vi "SCMP - rot180 array.vi"(7 "pic op (noop)":enum16{"noop", "Rot180", "Flip180"}(ring), 11 "A in":u32[][](array[numeric])) -> (3 "A out":u32[][](array[numeric]))   [LabVIEW 2014]
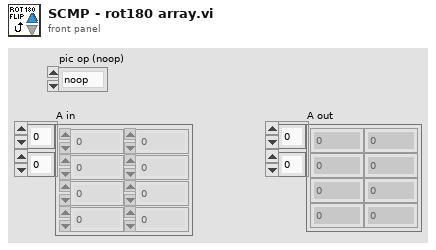
[diagram p1: front panel]
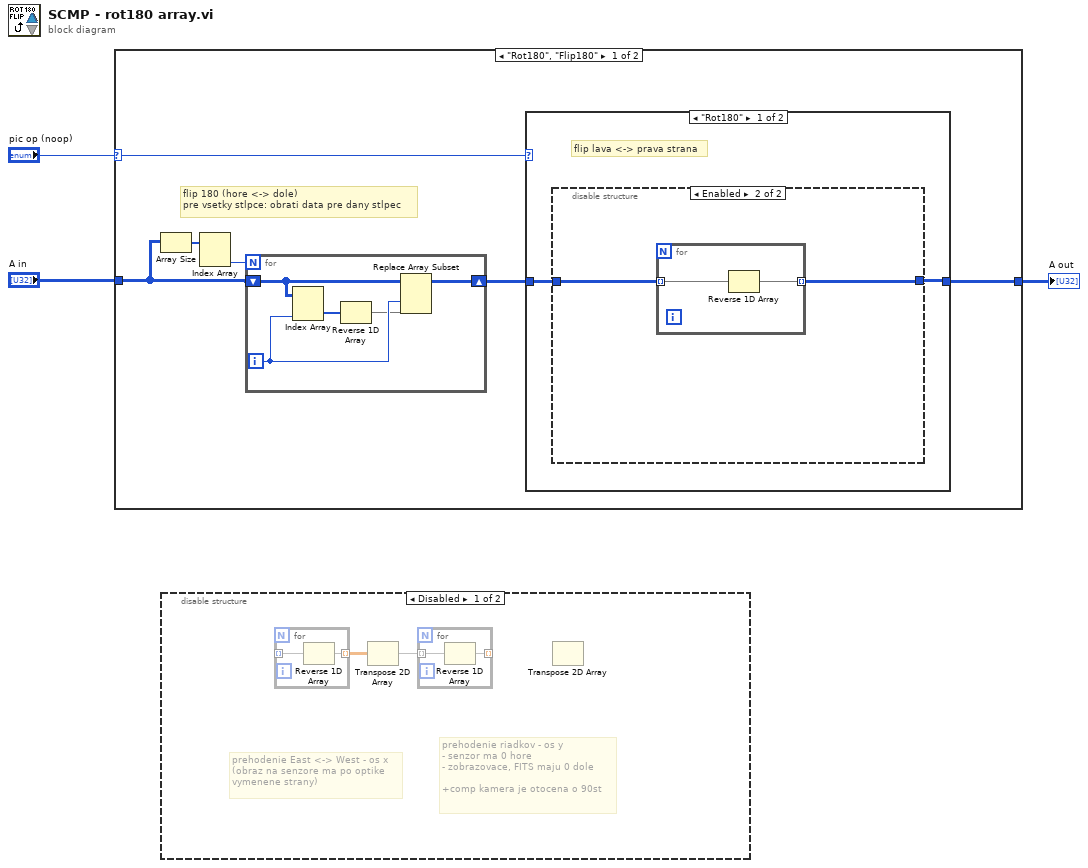
[diagram p0: block diagram]
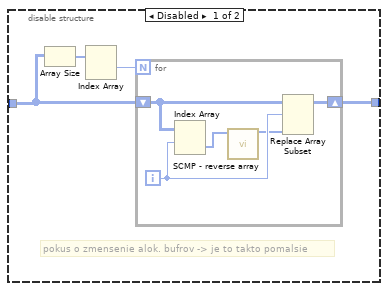
[diagram p3: hidden frame]
diagram:
  n1 = case shown="\"Rot180\", \"Flip180\"" "pic op (noop)" {
    selector: "pic op (noop)" -> [w5 _]
    tunnel: "A in" -> [w9 w31]
    tunnel: [w4 w31] -> w2
    frame "Rot180", "Flip180" {
      # "flip 180 (hore <-> dole)\npre vsetky stlpce: obrati data pre dany stlpec"
      n2 = Array Size(array=w9) -> (size(s)=w7:i32[])
      n3 = Index Array(array=w7) -> (element #2=w8:i32)  [unwired: 2 in, 1 out]
      n4 = for {
        N: w8 -> [_]
        shift-right: [w29] -> w6
        shift-left: w9 -> [w28]
        i -> [w30]
        n5 = Index Array(array=w28, index (col)=w30) -> (element=w27:u32[])  [unwired: 1 in]
        n6 = Reverse 1D Array(array=w27) -> (reversed array=w26:u32[])
        n7 = Replace Array Subset(array=w28, new element=w26, index (col)=w30) -> (w29:u32[][])  [unwired: 1 in]
      }
      n8 = case shown="\"Rot180\"" w5 {
        tunnel: w6 -> [w10 w25]
        tunnel: [w11 w25] -> w4
        frame "Rot180" {
          # "flip lava <-> prava strana"
          n9 = disable-structure shown="Enabled" {
            disable-tunnel: [w13 w21] -> w11
            disable-tunnel: w10 -> [w12 w22]
            frame Disabled {
              # "pokus o zmensenie alok. bufrov -> je to takto pomalsie"
              n10 = Array Size(array=w12) -> (size(s)=w15:i32[])
              n11 = Index Array(array=w15) -> (element #1=w14:i32)  [unwired: 2 in, 1 out]
              n12 = for {
                N: w14 -> [_]
                shift-right: [w19] -> w13
                shift-left: w12 -> [w18]
                i -> [w17]
                n13 = Index Array(array=w18, index (row)=w17) -> (element=w20:u32[])  [unwired: 1 in]
                n14 = call "SCMP - reverse array.vi"("A in"=w20) -> ("Array"=w16:u16[])  [unwired: 10 in]
                n15 = Replace Array Subset(array=w18, new element=w16, index (row)=w17) -> (w19:u32[][])  [unwired: 1 in]
              }
            }
            frame Enabled {
              n16 = for {
                tunnel: w22 -> [w24] mode=indexing
                tunnel: [w23] -> w21 mode=indexing
                n17 = Reverse 1D Array(array=w24) -> (reversed array=w23:u32[])
              }
            }
          }
        }
        frame "Flip180", Default {
        }
      }
    }
    frame "noop", Default {
    }
  }
  "A out" <- w2
  n18 = disable-structure shown="Disabled" {
    frame Disabled {
      # "prehodenie East <-> West - os x\n(obraz na senzore ma po optike \nvymenene strany)"
      # "prehodenie riadkov - os y\n- senzor ma 0 hore\n- zobrazovace, FITS maju 0 dole\n\n+comp kamera je otocena o 90st"
      n19 = for {
        tunnel: _ -> [w38] mode=indexing
        tunnel: [w37] -> w33 mode=indexing
        n20 = Reverse 1D Array(array=w38) -> (reversed array=w37:ext[])
      }
      n21 = Transpose 2D Array(2D array=w33) -> (transposed array=w32:ext[][])
      n22 = for {
        tunnel: w32 -> [w36] mode=indexing
        tunnel: [w35] -> _ mode=indexing
        n23 = Reverse 1D Array(array=w36) -> (reversed array=w35:ext[])
      }
      n24 = Transpose 2D Array() -> (2D array=w34:dbl[][])  [unwired: 1 out]
    }
    frame Enabled {
    }
  }
